vi "openVISA_current.vi"(6 "Boolean in":bool, 8 "error in (no error)":errorcluster, 11 "VISA Refnum in":refnum<visa-resource-name>) -> (0 "error out":errorcluster, 3 "VISA Refnum out":refnum<visa-resource-name>, 4 "Boolean out":bool)   [LabVIEW 2026]
uses:
  <vilib>/Instr/_visa.llb/VISA Configure Serial Port (Instr).vi
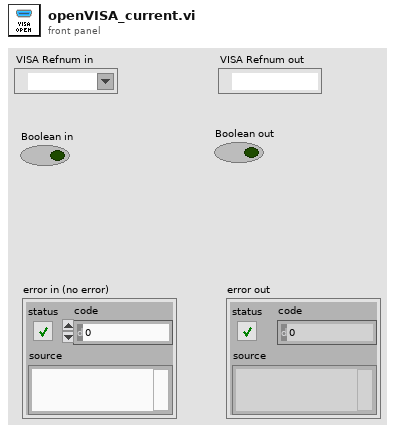
[diagram p1: front panel]
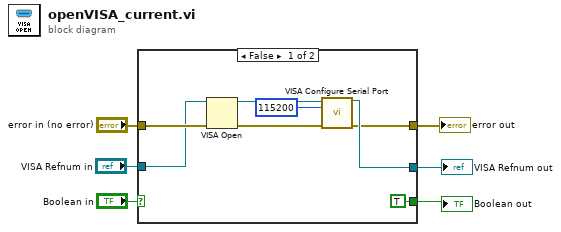
[diagram p0: block diagram]
diagram:
  n1 = case shown="False" "Boolean in" {
    selector: "Boolean in" -> [_ w17]
    tunnel: [TRUE w17] -> w3
    tunnel: "error in (no error)" -> [w9 w16]
    tunnel: [w11 w15] -> w5
    tunnel: [w10 w16] -> w6
    tunnel: "VISA Refnum in" -> [w7 w15]
    frame False {
      n2 = VISA Open(error in (no error)=w9, VISA resource name=w7) -> (VISA resource name=w13:refnum<visa-resource-name>, error out=w14:errorcluster)  [unwired: 3 in]
      n3 = call-poly "VISA Configure Serial Port"("VISA resource name"=w13, "baud rate (9600)"=u32 115200, "error in (no error)"=w14) -> ("VISA resource name out"=w11:refnum<visa-resource-name>, "error out"=w10:errorcluster)  [unwired: 11 in]
    }
    frame True {
    }
  }
  "error out" <- w6
  "VISA Refnum out" <- w5
  "Boolean out" <- w3
